vi "GUI_Highland.vi"() -> ()   [LabVIEW 2013]
uses:
  Shared/GUI_Template/GUI_master/tcp_new_data_event.ctl
  Shared/GUI_Template/GUI_master/tcp new data cluster.ctl
panel:
  out "tcp data event":T1
  in  "localsavingpath::1":path caption="LocalSavingPath"
  in  "channel4.width::1":dbl caption="Channel4.Width" min=0.0 max=10.0
  in  "channel4.delay::1":dbl caption="Channel4.Delay" min=0.0 max=10.0
  in  "channel4.polarity::1":enum16{"Direct", "Inverted"}(ring) caption="Channel4.Polarity"
  in  "channel4.channelon::1":enum16{"off", "on"}(ring) caption="Channel4.ChannelOn"
  in  "channel3.width::1":dbl caption="Channel3.Width" min=0.0 max=10.0
  in  "channel3.delay::1":dbl caption="Channel3.Delay" min=0.0 max=10.0
  in  "channel3.polarity::1":enum16{"Direct", "Inverted"}(ring) caption="Channel3.Polarity"
  in  "channel3.channelon::1":enum16{"off", "on"}(ring) caption="Channel3.ChannelOn"
  in  "channel2.width::1":dbl caption="Channel2.Width" min=0.0 max=10.0
  in  "channel2.delay::1":dbl caption="Channel2.Delay" min=0.0 max=10.0
  in  "channel2.polarity::1":enum16{"Direct", "Inverted"}(ring) caption="Channel2.Polarity"
  in  "channel2.channelon::1":enum16{"off", "on"}(ring) caption="Channel2.ChannelOn"
  in  "channel1.width::1":dbl caption="Channel1.Width" min=0.0 max=10.0
  in  "channel1.delay::1":dbl caption="Channel1.Delay" min=0.0 max=10.0
  in  "channel1.channelon::1":enum16{"off", "on"}(ring) caption="Channel1.ChannelOn"
  in  "channel1.polarity::1":enum16{"Direct", "Inverted"}(ring) caption="Channel1.Polarity"
  in  "trigger.source::1":T2(ring)=enum."Internal 80MHz" caption="Trigger.Source"
  in  "trigger.impedance::1":enum16{"10KOhm", "50Ohms"}(ring) caption="Trigger.Impedance"
  in  "trigger.divisor::1":dbl caption="Trigger.Divisor" min=1.0 max=9999.0
  in  "trigger.level::1":dbl caption="Trigger.Level" min=0.5 max=5.0
  out "UDP error message":string caption="Device Errors"
  in  "stop":bool
  in  "GUIdevice 1":string="HighlandT564DDG_Test(MM)"
  # "Channel parameters"
  # "Trigger Parameters"
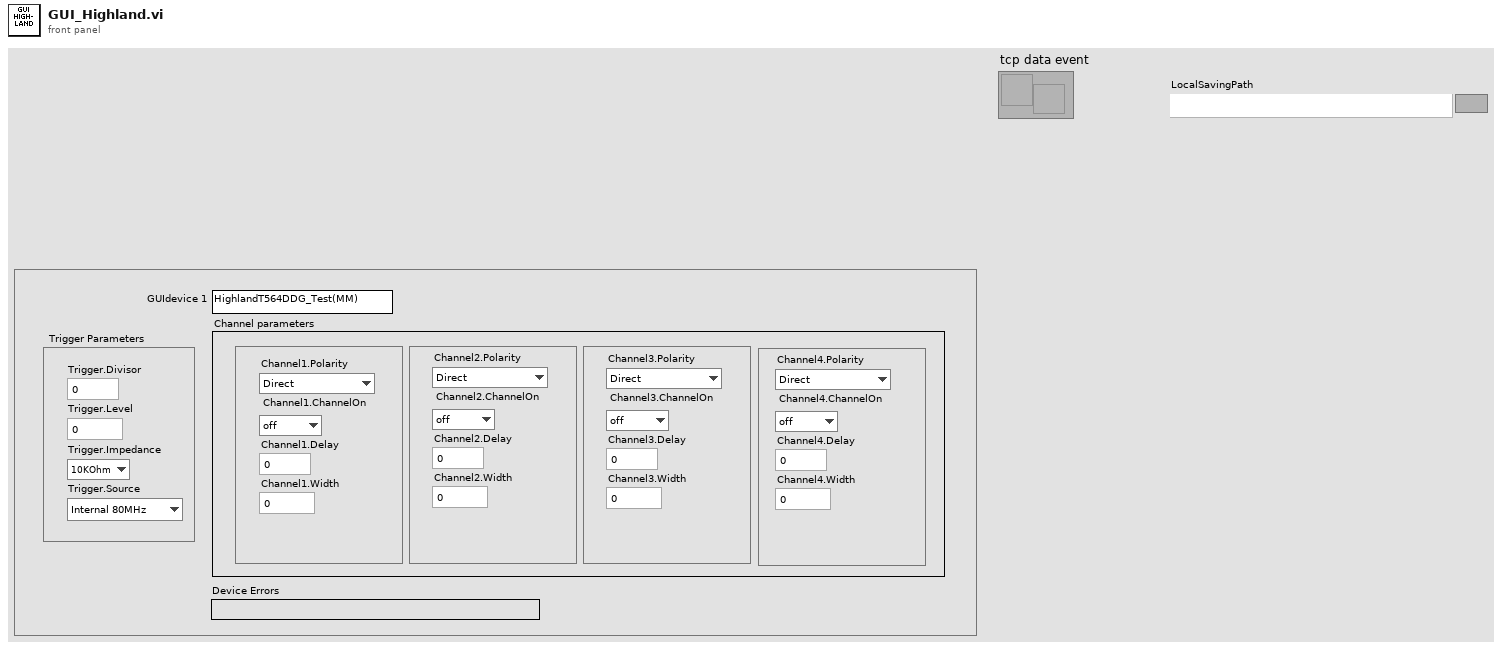
[diagram p1: front panel]
types:
  T1 = typedef "tcp_new_data_event.ctl" = refnum<user-event>
  T2 = enum16{"Rising", "Falling", "Internal 80MHz", "Internal DDS", "Remote", "Disabled"}
  T3 = enum32{"invalid app kind", "Development System", "Run Time System", "Student Edition", "Embedded LabVIEW", "Evaluation", "Custom"}
  T4 = typedef "tcp new data cluster.ctl" = cluster{"EventEnum":enum16{"new data", "connection status update"}, "Device name":string}
  T5 = enum32{"Invalid", "Standard", "Closed", "Hidden", "Minimized", "Maximized"}
  T6 = cluster{"Core":cluster{"Current VI Reference":refnum<vi>, "Close Panel on Exit?":bool}, "Your Boolean data":bool, "Your string data":string, "SuperGUI":cluster{"STOP queue":refnum<queue>, "SuperGUI ref":refnum<vi>}}
  T7 = cluster{"STOP queue":refnum<queue>, "SuperGUI ref":refnum<vi>}
  T8 = cluster{"Current VI Reference":refnum<vi>, "Close Panel on Exit?":bool}
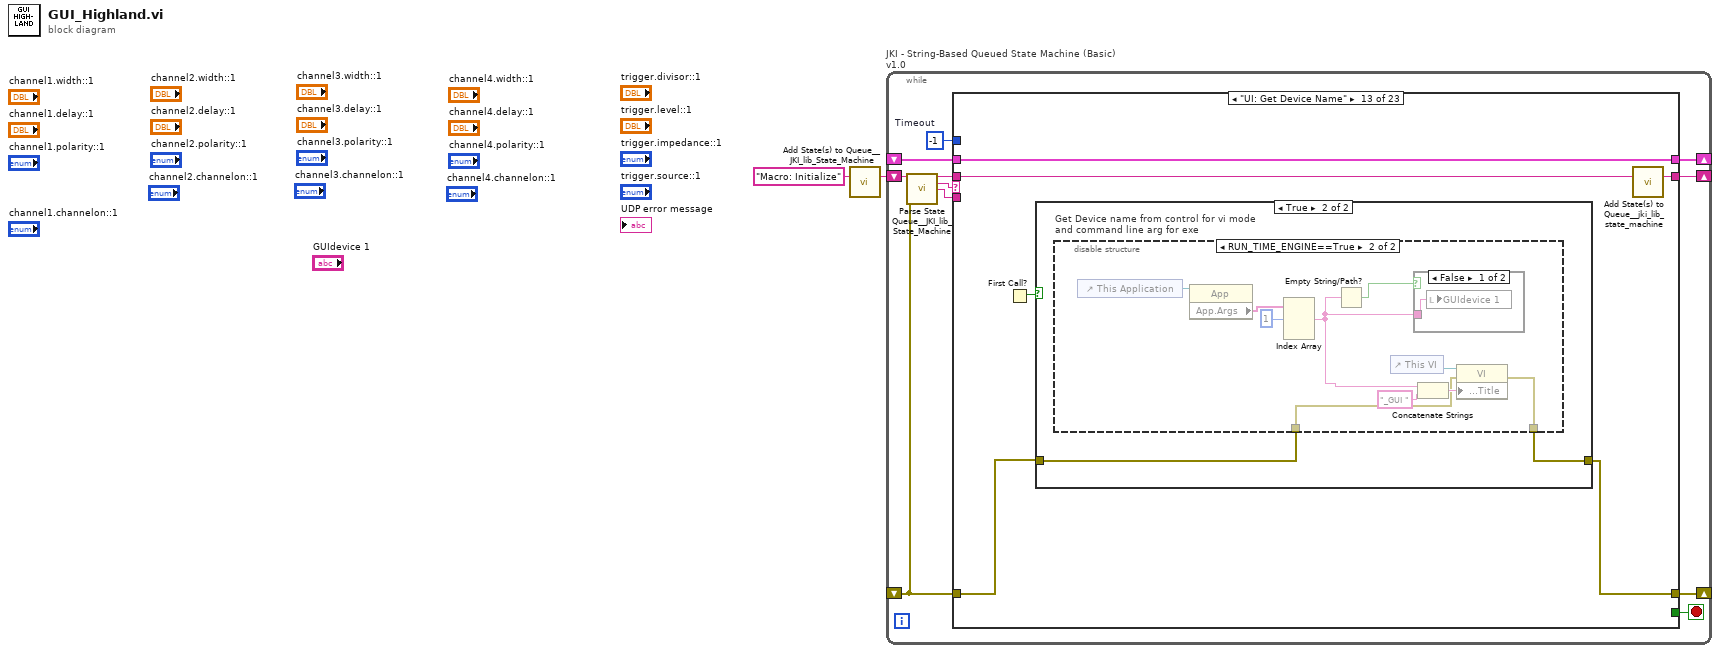
[diagram p0: block diagram]
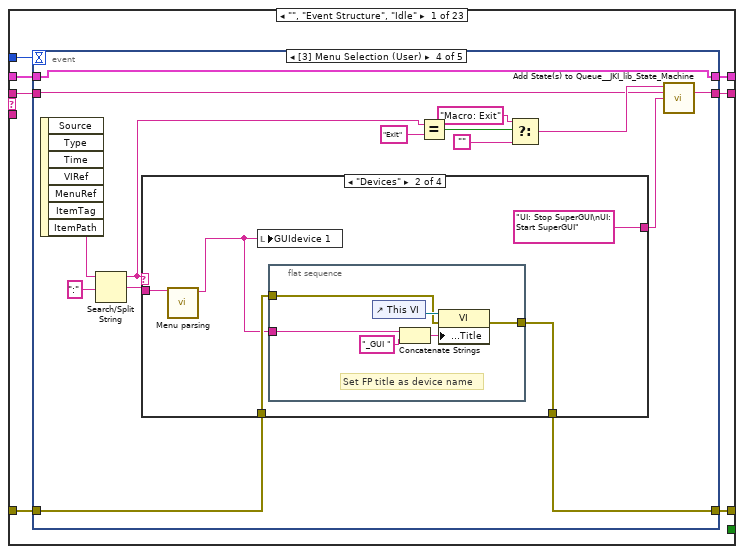
[diagram p2: hidden frame]
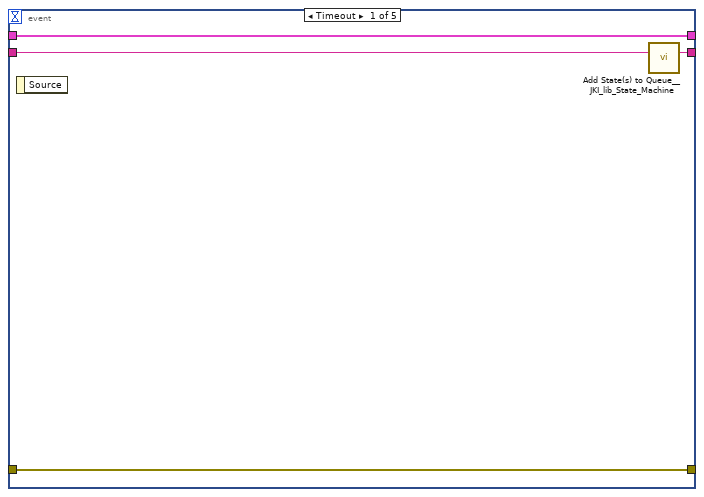
[diagram p3: hidden frame]
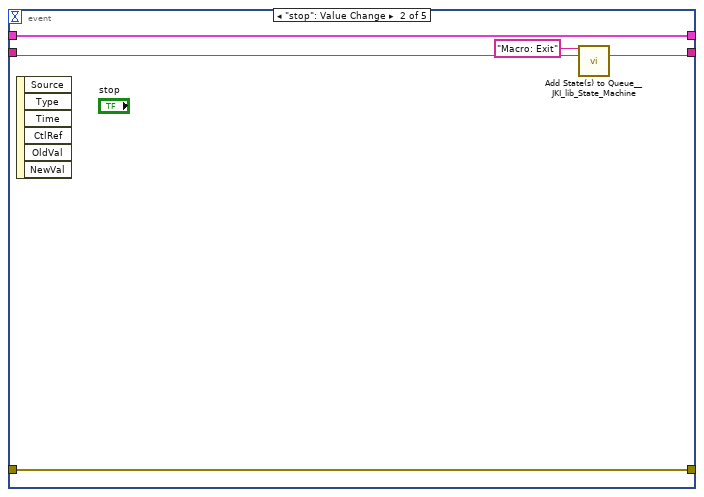
[diagram p4: hidden frame]
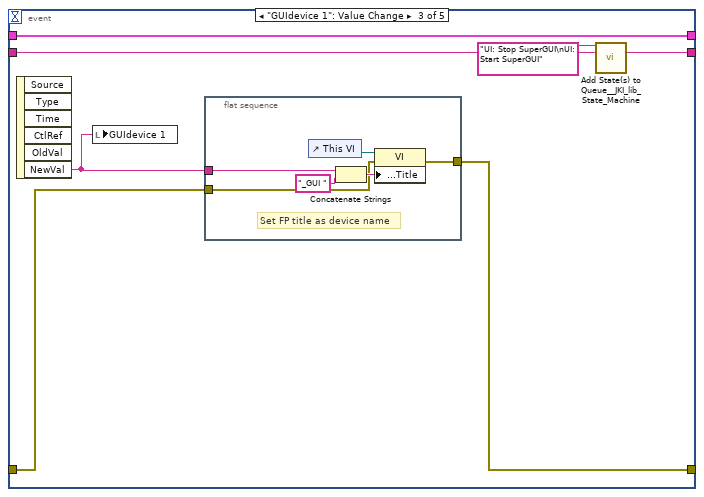
[diagram p5: hidden frame]
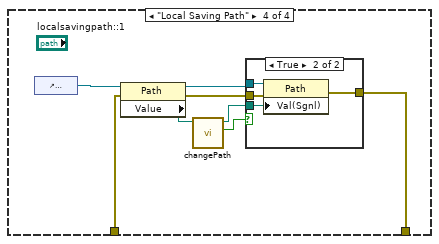
[diagram p8: hidden frame]
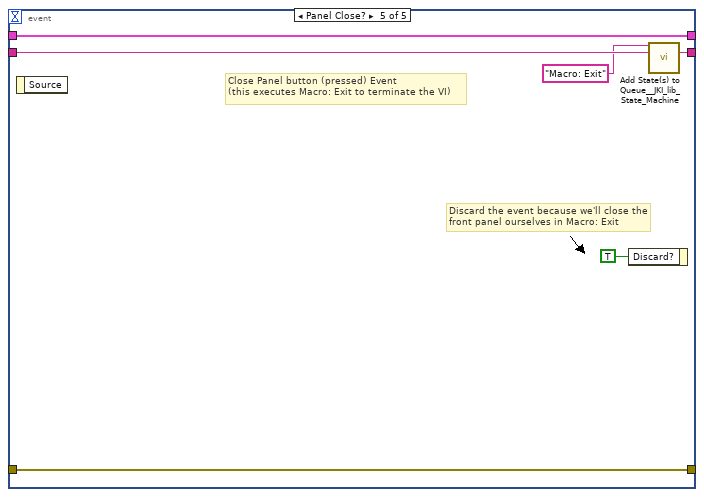
[diagram p10: hidden frame]
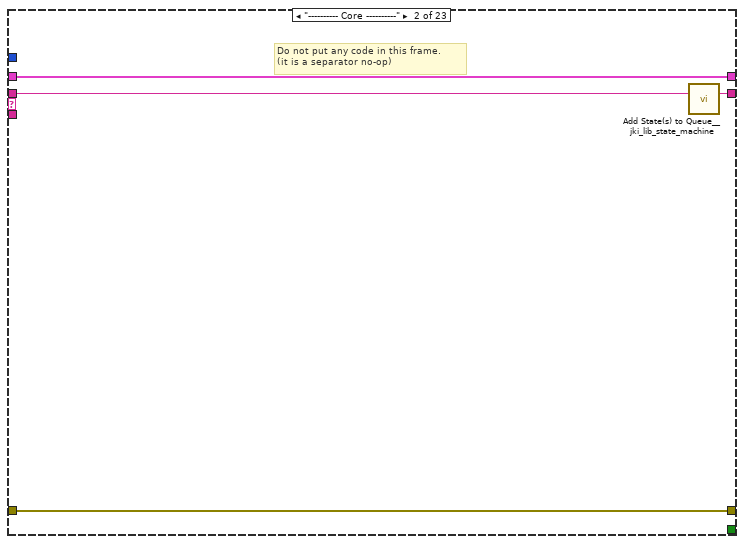
[diagram p11: hidden frame]
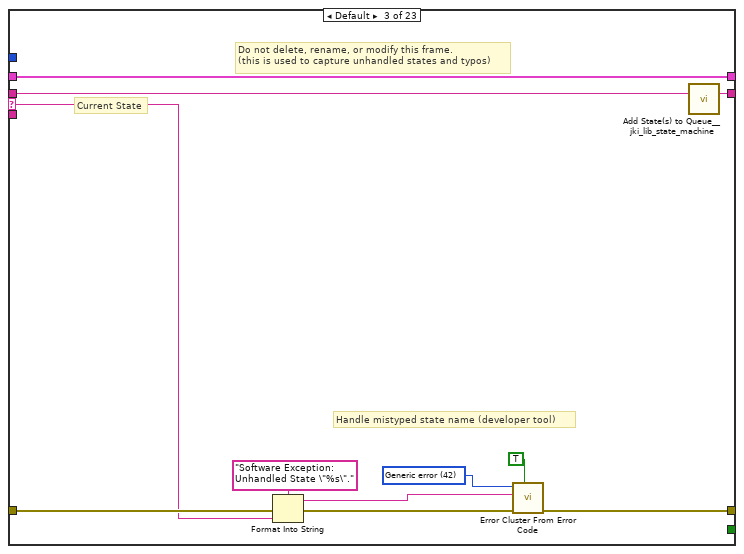
[diagram p12: hidden frame]
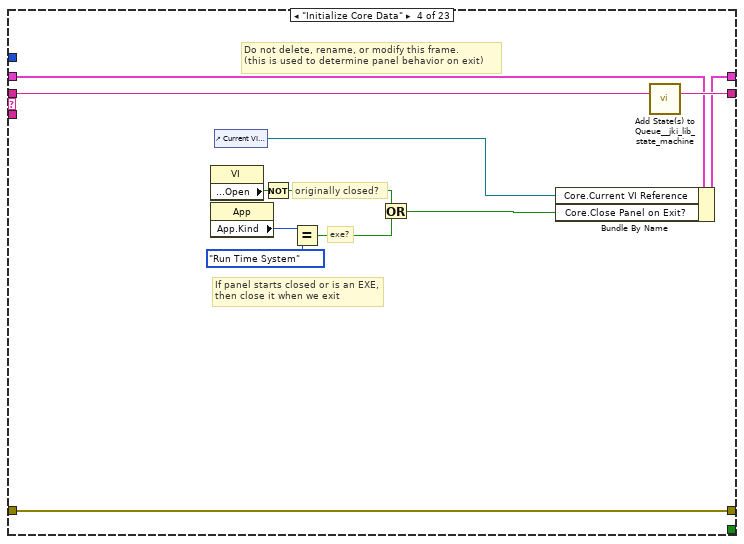
[diagram p13: hidden frame]
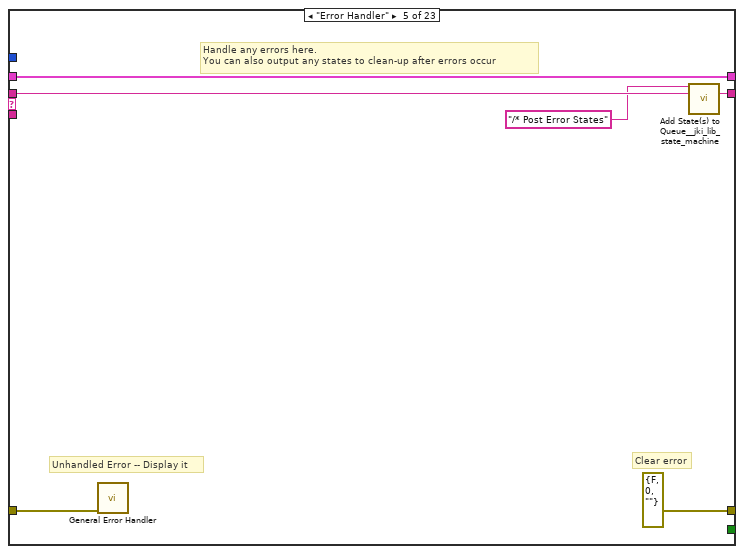
[diagram p14: hidden frame]
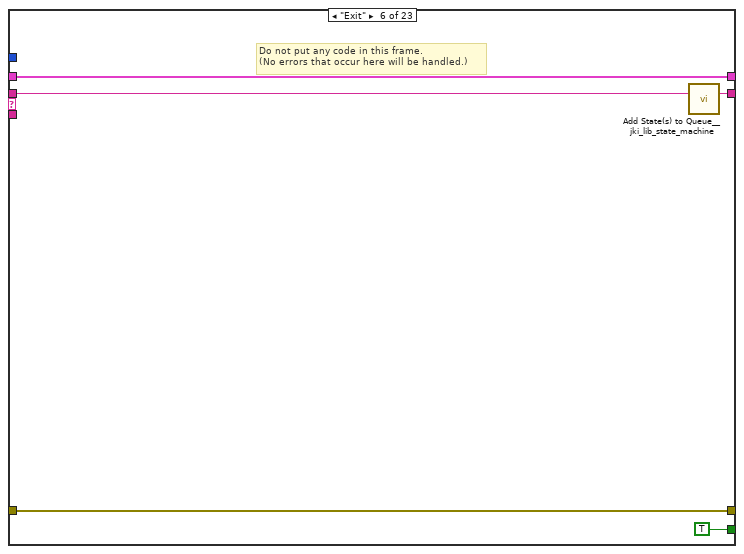
[diagram p15: hidden frame]
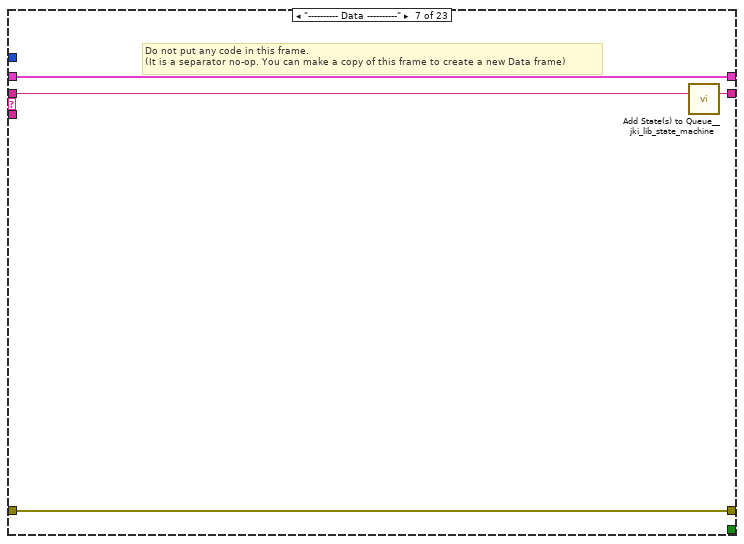
[diagram p16: hidden frame]
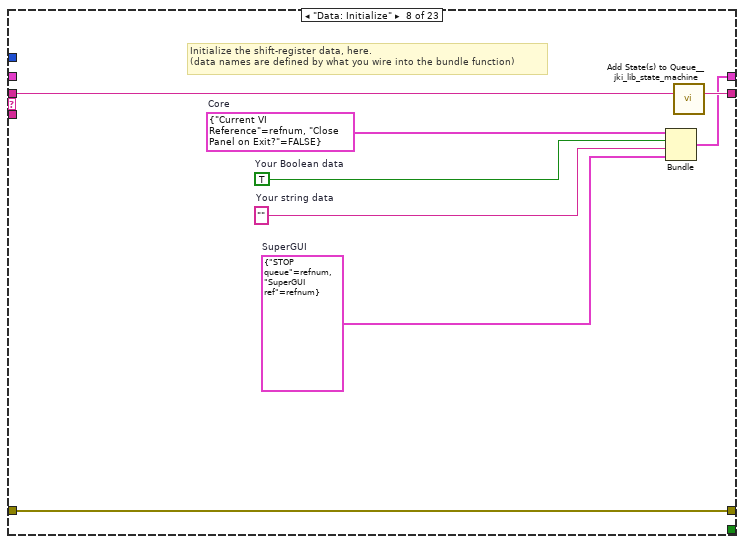
[diagram p17: hidden frame]
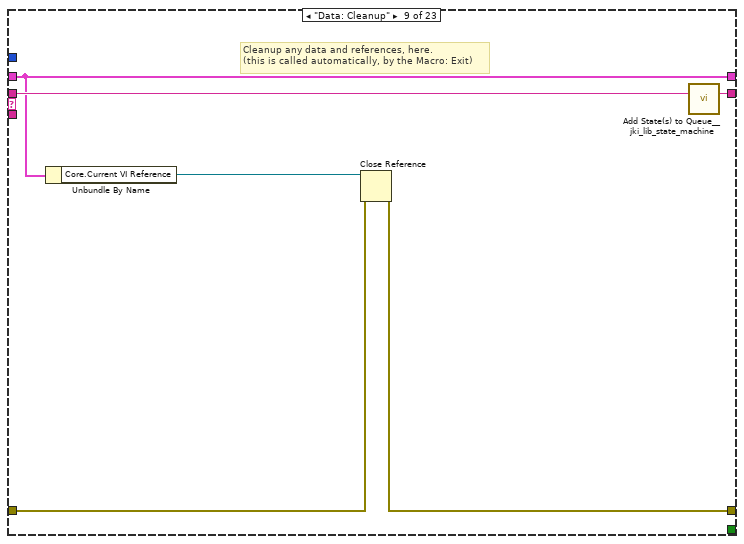
[diagram p18: hidden frame]
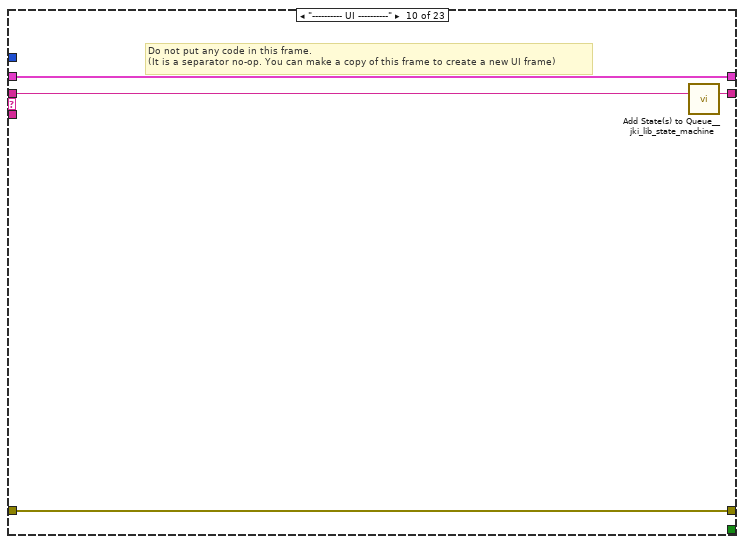
[diagram p19: hidden frame]
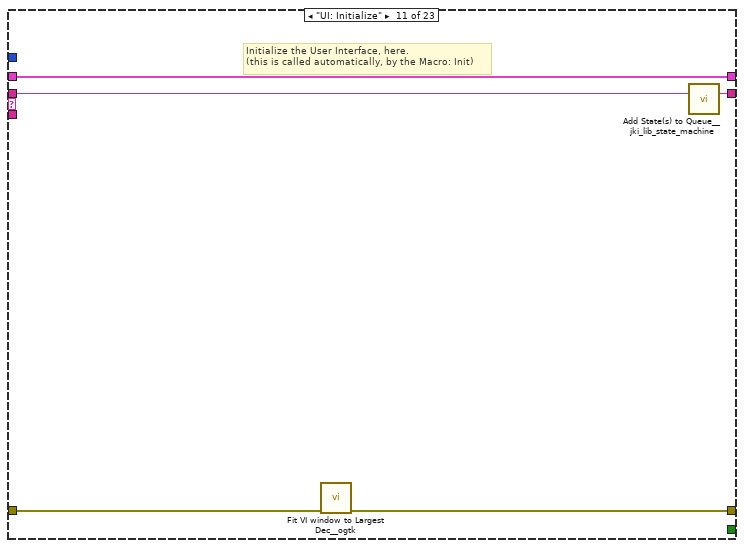
[diagram p20: hidden frame]
diagram:
  n1 = call <vilib>:"Add State(s) to Queue__JKI_lib_State_Machine.vi"("State(s) in (\"\")"="Macro: Initialize") -> ("States Out"=w2:string)  [unwired: 14 in]
  n2 = while "JKI - String-Based Queued State Machine (Basic) v1.0" {
    shift-right: [w6] -> _
    shift-left: _ -> [w5]
    shift-right: [w9] -> _
    shift-left: _ -> [w3]
    shift-right: [w8] -> _
    shift-left: w2 -> [w10]
    stop <- w7 stop-if-true
    w4 = -1  # Timeout
    n3 = call <vilib>:"Parse State Queue__JKI_lib_State_Machine.vi"("State Queue"=w10, "Error In (no error)"=w3) -> ("Remaining States"=w12:string, "Current State"=w13:string, "Arguments"=w11:string)  [unwired: 11 in]
    n4 = case shown="\"UI: Get Device Name\"" w13 {
      selector: w13 -> [_ _ w94 _ _ _ _ _ _ _ _ _ _ _ _ _ _ _ _ _ _ _ _]
      tunnel: w12 -> [w20 w93 w98 w116 w122 w127 w131 w139 w145 w149 w154 w162 w194 w228 w236 w242 w253 w279 w284 w294 w298 w302 w306]
      tunnel: w11 -> [_ _ _ _ _ _ _ _ _ _ _ _ _ _ _ w237 w247 _ _ _ _ _ _]
      tunnel: w5 -> [w18 w90 w96 w107 w119 w125 w128 _ w140 w146 w152 w160 w192 w219 w231 w240 w249 w276 w281 w291 w295 w299 w303]
      tunnel: [w17 w91 w100 w113 errorcluster {"status"=FALSE, "code"=0, "source"=""} ("error out") w124 w129 w136 w141 w147 w150 w158 w189 w212 w229 w238 w250 w277 w282 w292 w296 w300 w304] -> w9
      tunnel: w3 -> [w16 w91 w99 w113 w118 w124 w129 w136 w142 w147 w151 w159 w190 w213 w230 w239 w251 w277 w282 w292 w296 w300 w304]
      tunnel: [w19 w92 w97 w115 w121 w126 w130 w138 w144 w148 w153 w161 w193 w227 w235 w241 w252 w278 w283 w293 w297 w301 w305] -> w8
      tunnel: [_ _ _ _ _ TRUE _ _ _ _ _ _ _ _ _ _ _ _ _ _ _ _ _] -> w7
      tunnel: [w15 w90 w96 w114 w119 w125 w128 w137 w140 w146 w152 w160 w192 w218 w231 w240 w249 w276 w281 w291 w295 w299 w303] -> w6
      tunnel: w4 -> [w14 _ _ _ _ _ _ _ _ _ _ _ _ _ _ _ _ _ _ _ _ _ _]
      frame "", "Event Structure", "Idle" {
        n5 = event shown="[3] Menu Selection (User)" {
          selector: _ -> [_ _ _ _ _]
          dyn-events: _ -> [_ _ _ _ _]
          timeout: w14 -> [_ _ _ _ _]
          tunnel: w20 -> [w24 w27 w33 w51 w89]
          tunnel: [w23 w26 w32 w50 w88] -> w19
          tunnel: w18 -> [w21 w29 w36 w57 w86]
          tunnel: [w22 w28 w34 w44 w87] -> w17
          tunnel: w16 -> [w22 w28 w35 w45 w87]
          tunnel: [w21 w29 w36 w57 w86] -> w15
          event Timeout {
            n6 = event-data() -> ()  [unwired: 1 in, 1 out]
            n7 = call <vilib>:"Add State(s) to Queue__JKI_lib_State_Machine.vi"("State(s) in (\"\")"=w24) -> ("States Out"=w23:string)  [unwired: 14 in]
          }
          event "stop": Value Change {
            n8 = event-data() -> ()  [unwired: 1 in, 6 out]
            n9 = call <vilib>:"Add State(s) to Queue__JKI_lib_State_Machine.vi"("State(s) in Front (\"\")"="Macro: Exit", "State(s) in (\"\")"=w27) -> ("States Out"=w26:string)  [unwired: 13 in]
          }
          event "GUIdevice 1": Value Change {
            n10 = event-data() -> ("NewVal"=w30:string)  [unwired: 1 in, 5 out]
            n11 = local write "GUIdevice 1"(w30) -> ()
            n12 = flat-sequence {
              tunnel: [w39] -> w34
              tunnel: w35 -> [w38]
              tunnel: w30 -> [w37]
              frame #0 {
                # "Set FP title as device name"
                n13 = control-ref of="This VI"() -> (w42:refnum<vi>)
                n14 = Concatenate Strings(w37, "_GUI ") -> (w41:string)
                n15 = property class="VI"(reference=w42, error in=w38, "Front Panel.Title"=w41) -> (error out=w39:errorcluster)  [unwired: 1 out]
              }
            }
            n16 = call <vilib>:"Add State(s) to Queue__JKI_lib_State_Machine.vi"("State(s) in Front (\"\")"="UI: Stop SuperGUI\nUI: Start SuperGUI", "State(s) in (\"\")"=w33) -> ("States Out"=w32:string)  [unwired: 13 in]
          }
          event Menu Selection (User) {
            n17 = event-data() -> ("ItemPath"=w47:string)  [unwired: 1 in, 6 out]
            n18 = Search/Split String(string=w47, search string/char (-)=":") -> (substring before match=w43:string, match + rest of string=w46:string)  [unwired: 1 in, 1 out]
            n19 = case shown="\"Devices\"" w43 {
              tunnel: w46 -> [_ w63 _ _]
              tunnel: w45 -> [w58 w62 w70 w73]
              tunnel: [w58 w61 w70 w72] -> w44
              tunnel: [_ "UI: Stop SuperGUI\nUI: Start SuperGUI" _ _] -> w49
              frame "", Default {
              }
              frame "Devices" {
                n20 = call "Menu parsing.vi"("ItemPath"=w63) -> ("ItemPath"=w59:string)  [unwired: 9 in, 1 out]
                n21 = local write "GUIdevice 1"(w59) -> ()
                n22 = flat-sequence {
                  tunnel: [w66] -> w61
                  tunnel: w62 -> [w65]
                  tunnel: w59 -> [w64]
                  frame #0 {
                    # "Set FP title as device name"
                    n23 = control-ref of="This VI"() -> (w69:refnum<vi>)
                    n24 = Concatenate Strings(w64, "_GUI ") -> (w68:string)
                    n25 = property class="VI"(reference=w69, error in=w65, "Front Panel.Title"=w68) -> (error out=w66:errorcluster)  [unwired: 1 out]
                  }
                }
              }
              frame "Exit" {
              }
              frame "Local Saving Path" {
                n26 = control-ref of="localsavingpath::1"() -> (w74:refnum<vi>)
                n27 = property class="Path"(reference=w74, error in=w73) -> (reference out=w76:refnum<vi>, error out=w71:errorcluster, "Value"=w75:path)
                n28 = call "changePath.vi"("Local Saving in (h)"=w75) -> ("change (h)"=w77:bool, "Local Saving out (h)"=w78:path)  [unwired: 9 in]
                n29 = case shown="True" w77 {
                  tunnel: w76 -> [_ w83]
                  tunnel: w78 -> [_ w82]
                  tunnel: [w79 w81] -> w72
                  tunnel: w71 -> [w79 w80]
                  frame False {
                  }
                  frame True {
                    n30 = property class="Path"(reference=w83, error in=w80, "Val(Sgnl)"=w82) -> (error out=w81:errorcluster)  [unwired: 1 out]
                  }
                }
              }
            }
            n31 = Equal?(x=w43, y="Exit") -> (x = y?=w55:bool)
            n32 = Select(t="Macro: Exit", s=w55, f="") -> (s? t:f=w52:string)
            n33 = call <vilib>:"Add State(s) to Queue__JKI_lib_State_Machine.vi"("State(s) in Front (\"\")"=w52, "State(s) in (\"\")"=w51, "State(s) at Back (\"\")"=w49) -> ("States Out"=w50:string)  [unwired: 12 in]
          }
          event Panel Close? {
            # "Discard the event because we'll close the front panel ourselves in Macro: Exit"
            # "Close Panel button (pressed) Event\n(this executes Macro: Exit to terminate the VI)"
            n34 = event-data() -> ()  [unwired: 1 in, 1 out]
            n35 = event-data("Discard?"=TRUE) -> ()  [unwired: 1 in, 1 out]
            n36 = call <vilib>:"Add State(s) to Queue__JKI_lib_State_Machine.vi"("State(s) in Front (\"\")"="Macro: Exit", "State(s) in (\"\")"=w89) -> ("States Out"=w88:string)  [unwired: 13 in]
          }
        }
      }
      frame "---------- Core ----------" {
        # "Do not put any code in this frame.\n(it is a separator no-op)"
        n37 = call <vilib>:"Add State(s) to Queue__jki_lib_state_machine.vi"("State(s) in (\"\")"=w93) -> ("States Out"=w92:string)  [unwired: 14 in]
      }
      frame Default {
        w103 = 42 items=["No error", "Argument error", "Memory is full", "Out of zone", "End of file", "File already open", "Generic file I/O error", "File not found", "File permission error", "Disk is full", "Duplicate path", "Too many files open", "System feature not enabled", "Resource file not found", "Cannot add resource", "Resource not found", "Image not found", "Image memory error", "Pen does not exist", "Config type invalid", "Config token not found", "Config parse error", "Config memory error", "Bad external code format", "Bad external code offset", "External code not present", "Null window", "Destroy window error", "Null menu", "Print aborted", "Bad print record", "Print driver error", "Windows error during printing", "Memory error during printing", "Print dialog error", "Generic print error", "Invalid device refnum", "Device not found", "Device parameter error", "Device unit error", "Cannot open device", "Device call aborted", "Generic error", "Cancelled by user", "Object ID too low", "Object ID too high", "Object not in heap", "Unknown heap", "Unknown object (invalid DefProc)", "Unknown object (DefProc not in table)", "Message out of range", "Invalid (null) method", "Unknown message", "Manager call not supported", "Bad address", "Network operation in progress", "Network operation timed out", "Connection is busy", "Network attribute not supported", "Network error", "Address in use", "System out of memory", "Connection aborted", "Connection refused", "Not connected", "Already connected", "Connection closed", "Initialization error (interapplication manager)", "Bad occurrence", "Wait on unbound occurrence handler", "Occurrence queue overflow", "Datalog type conflict", "Unused", "Unrecognized type (interapplication manager)", "Memory corrupt", "Failed to make temporary DLL", "Old CIN version", "Drag socket not found", "Failed to load drop-object", "Failed to register OLE object", "Failed to release OLE object", "Format specifier type mismatch", "Unknown format specifier", "Too few format specifiers", "Too many format specifiers", "Scan failed", "Newer CIN version", "Error converting to variant", "Runtime menu error", "Password tampered", "Variant attribute not found", "Incompatible variant data type", "Event data is not available", "Event Store is not present", "Occurrence is not found", "Event Queue is not created", "Event info is not available", "Refnum passed is NULL", "Error retrieving Class GUID", "Error retrieving CoClass GUID", "Error retrieving TypeLib GUID.", "Bad built application magic bytes.", "Specific driver is different from the specific driver associated with the Logical Name.", "There is no session opened to the class driver.", "Max Error", "MAX - Error with config objects", "MAX - Error loading configuration", "MAX - Group not supported"]
        # "Current State"
        # "Do not delete, rename, or modify this frame.\n(this is used to capture unhandled states and typos)"
        # "Handle mistyped state name (developer tool)"
        n38 = Format Into String(format string="Software Exception: Unhandled State \"%s\"." ("message"), error in=w99, w94) -> (resulting string=w102:string, error out=w101:errorcluster)  [unwired: 1 in]
        n39 = call <vilib>:"Error Cluster From Error Code.vi"("show call chain? (False)"=TRUE, "error in (no error)"=w101, "error message (\"\")"=w102, "error code (0)"=w103) -> ("error out"=w100:errorcluster)  [unwired: 5 in]
        n40 = call <vilib>:"Add State(s) to Queue__jki_lib_state_machine.vi"("State(s) in (\"\")"=w98) -> ("States Out"=w97:string)  [unwired: 14 in]
      }
      frame "Initialize Core Data" {
        # "Do not delete, rename, or modify this frame.\n(this is used to determine panel behavior on exit)"
        # "originally closed?"
        # "exe?"
        # "If panel starts closed or is an EXE, then close it when we exit"
        n41 = property class="VI"() -> ("Front Panel.Open"=w112:bool)  [unwired: 2 in, 2 out]
        n42 = property class="App"() -> ("App.Kind"=w111:T3)  [unwired: 2 in, 2 out]
        n43 = control-ref of="Current VI Reference"() -> (w105:refnum<vi>)
        n44 = Not(x=w112) -> (.not. x?=w109:bool)
        n45 = Equal?(x=w111, y=T3."Run Time System" ("Application:Kind")) -> (x = y?=w108:bool)
        n46 = Or(x=w109, y=w108) -> (x .or. y?=w106:bool)
        n47 = Bundle By Name(cluster=w107, "Core.Current VI Reference"=w105, "Core.Close Panel on Exit?"=w106) -> (w114:T6)
        n48 = call <vilib>:"Add State(s) to Queue__jki_lib_state_machine.vi"("State(s) in (\"\")"=w116) -> ("States Out"=w115:string)  [unwired: 14 in]
      }
      frame "Error Handler" {
        # "Unhandled Error -- Display it"
        # "Handle any errors here.\nYou can also output any states to clean-up after errors occur"
        # "Clear error"
        n49 = call <vilib>:"General Error Handler.vi"("error in (no error)"=w118) -> ()  [unwired: 10 in, 5 out]
        n50 = call <vilib>:"Add State(s) to Queue__jki_lib_state_machine.vi"("State(s) in Front (\"\")"="/* Post Error States", "State(s) in (\"\")"=w122) -> ("States Out"=w121:string)  [unwired: 13 in]
      }
      frame "Exit" {
        # "Do not put any code in this frame.\n(No errors that occur here will be handled.)"
        n51 = call <vilib>:"Add State(s) to Queue__jki_lib_state_machine.vi"("State(s) in (\"\")"=w127) -> ("States Out"=w126:string)  [unwired: 14 in]
      }
      frame "---------- Data ----------" {
        # "Do not put any code in this frame.\n(It is a separator no-op. You can make a copy of this frame to create a new Data frame)"
        n52 = call <vilib>:"Add State(s) to Queue__jki_lib_state_machine.vi"("State(s) in (\"\")"=w131) -> ("States Out"=w130:string)  [unwired: 14 in]
      }
      frame "Data: Initialize" {
        w132 = T7 {"STOP queue"=refnum, "SuperGUI ref"=refnum}  # SuperGUI
        w133 = T8 {"Current VI Reference"=refnum, "Close Panel on Exit?"=FALSE}  # Core
        w135 = TRUE  # Your Boolean data
        w134 = ""  # Your string data
        # "Initialize the shift-register data, here.\n(data names are defined by what you wire into the bundle function)"
        n53 = Bundle("Core"=w133, "Your Boolean data"=w135, "Your string data"=w134, "SuperGUI"=w132) -> (w137:T6)  [unwired: 1 in]
        n54 = call <vilib>:"Add State(s) to Queue__jki_lib_state_machine.vi"("State(s) in (\"\")"=w139) -> ("States Out"=w138:string)  [unwired: 14 in]
      }
      frame "Data: Cleanup" {
        # "Cleanup any data and references, here.\n(this is called automatically, by the Macro: Exit)"
        n55 = Unbundle By Name(w140) -> ("Core.Current VI Reference"=w143:refnum<vi>)
        n56 = Close Reference(reference=w143, error in (no error)=w142) -> (error out=w141:errorcluster)
        n57 = call <vilib>:"Add State(s) to Queue__jki_lib_state_machine.vi"("State(s) in (\"\")"=w145) -> ("States Out"=w144:string)  [unwired: 14 in]
      }
      frame "---------- UI ----------" {
        # "Do not put any code in this frame.\n(It is a separator no-op. You can make a copy of this frame to create a new UI frame)"
        n58 = call <vilib>:"Add State(s) to Queue__jki_lib_state_machine.vi"("State(s) in (\"\")"=w149) -> ("States Out"=w148:string)  [unwired: 14 in]
      }
      frame "UI: Initialize" {
        # "Initialize the User Interface, here.\n(this is called automatically, by the Macro: Init)"
        n59 = call <userlib>:"Fit VI window to Largest Dec__ogtk.vi"("error in (no error)"=w151) -> ("error out"=w150:errorcluster)  [unwired: 5 in, 1 out]
        n60 = call <vilib>:"Add State(s) to Queue__jki_lib_state_machine.vi"("State(s) in (\"\")"=w154) -> ("States Out"=w153:string)  [unwired: 14 in]
      }
      frame "UI: Update Device List" {
        n61 = call "getDevices.vi"("Device Class"="Highland T564 DDG") -> ("All Devices"=w156:string[])
        n62 = Empty Array?(array=w156) -> (empty?=w157:bool)
        n63 = case shown="False" w157 {
          tunnel: w159 -> [w165 w188]
          tunnel: [w164 w188] -> w158
          tunnel: w156 -> [w163 _]
          frame False {
            n64 = Current VI's Menubar() -> (w168:refnum<k9>)
            n65 = Get Menu Item Info(7:"Devices" ("item tag"), 8:w165, 11:w168) -> (0:w174:errorcluster, 3:w170:refnum<k9>)  [unwired: 5 out]
            n66 = Set Menu Item Info(7:"Devices" ("item tag"), 8:w174, 9:TRUE ("enabled"), 11:w170) -> (0:w173:errorcluster, 3:w172:refnum<k9>)  [unwired: 3 in]
            n67 = First Call?() -> (First Call?: T/F=w166:bool)
            n68 = case shown="True" w166 {
              tunnel: w172 -> [_ w180]
              tunnel: w163 -> [_ w179]
              tunnel: w173 -> [w175 w177]
              tunnel: [w175 w176] -> w164
              frame False {
              }
              frame True {
                n69 = for {
                  tunnel: [w187] -> w181
                  tunnel: w179 -> [w185] mode=indexing
                  tunnel: w180 -> [w184]
                  tunnel: [w183] -> w178
                  tunnel: w177 -> [w182]
                  n70 = Insert Menu Items(5:"Devices" ("menu tag"), 6:w182, 7:w185, 8:w185, 9:w184) -> (0:w183:errorcluster, 3:w187:refnum<k9>)  [unwired: 1 in, 1 out]
                }
                n71 = Enable Menu Tracking(2:w178, 4:w181) -> (0:w176:errorcluster)  [unwired: 1 in, 1 out]
              }
            }
          }
          frame True {
          }
        }
        n72 = call <vilib>:"Add State(s) to Queue__jki_lib_state_machine.vi"("State(s) in (\"\")"=w162) -> ("States Out"=w161:string)  [unwired: 14 in]
      }
      frame "UI: Get Device Name" {
        n73 = First Call?() -> (First Call?: T/F=w191:bool)
        n74 = case shown="True" w191 {
          tunnel: w190 -> [w195 w197]
          tunnel: [w195 w196] -> w189
          frame False {
          }
          frame True {
            n75 = disable-structure "Get Device name from control for vi mode\nand command line arg for exe" shown="RUN_TIME_ENGINE==True" {
              disable-tunnel: w197 -> [_ w199]
              disable-tunnel: [_ w198] -> w196
              frame condition #0 (active) {
              }
              frame condition #1 {
                n76 = control-ref of="This Application"() -> (w207:refnum<vi>)
                n77 = property class="App"(reference=w207) -> ("App.Args"=w206:string[])  [unwired: 1 in, 2 out]
                n78 = Index Array(array=w206, index #1=1 ("index")) -> (element #1=w200:string)  [unwired: 2 in, 2 out]
                n79 = Empty String/Path?(string/path=w200) -> (empty?=w204:bool)
                n80 = control-ref of="This VI"() -> (w203:refnum<vi>)
                n81 = case shown="False" w204 {
                  tunnel: w200 -> [w208 _]
                  frame False {
                    n82 = local write "GUIdevice 1"(w208) -> ()
                  }
                  frame True {
                  }
                }
                n83 = Concatenate Strings(w200, "_GUI ") -> (w202:string)
                n84 = property class="VI"(reference=w203, error in=w199, "Front Panel.Title"=w202) -> (error out=w198:errorcluster)  [unwired: 1 out]
              }
            }
          }
        }
        n85 = call <vilib>:"Add State(s) to Queue__jki_lib_state_machine.vi"("State(s) in (\"\")"=w194) -> ("States Out"=w193:string)  [unwired: 14 in]
      }
      frame "UI: Start SuperGUI" {
        # "create stop queue for supergui and its clones"
        # "x100 abort will be dependent on caller VI\nx80 abort will be independent of caller vi, this will abort vi when labview is closed."
        # "Start SuperGUI asynchronous way"
        n86 = vi-ref "GUI_Master_subvi_reentrant_queues.vi"() -> (w211:refnum<vi>)
        n87 = property class="VI"(reference=w211) -> ("Path"=w210:path)  [unwired: 1 in, 2 out]
        n88 = Create User Event(user event datatype=T4 {"EventEnum"=enum."new data", "Device name"="Device name"} ("New Event"), error in=w213) -> (user event=w214:refnum<user-event>, error out=w220:errorcluster)
        "tcp data event" <- w214
        n89 = control-ref of="This Application"() -> (w217:refnum<vi>)
        n90 = control-ref of="This VI"() -> (w216:refnum<vi>)
        n91 = Open VI Reference(type specifier VI Refnum (for type only)=refnum<vi> refnum, vi path=w210, options=256) -> (vi reference=w226:refnum<vi>, error out=w225:errorcluster)  [unwired: 3 in]
        n92 = register-events(w214) -> ()  [unwired: 2 in, 2 out]
        n93 = call "supergui create stop queue.vi"() -> ("STOP Queue out"=w222:refnum<queue>)  [unwired: 11 in]
        n94 = Current VI's Menubar() -> (w215:refnum<k9>)
        n95 = call-by-ref "Start Asynchronous Call"(reference=w226, error in=w225, "STOP Queue in"=w222, "This Application"=w217, 8:"error in (no error)"=w220, "tcp data event"=w214, "Caller menu reference"=w215, "Caller VI ref"=w216) -> (reference out=w209:refnum<vi>, error out=w212:errorcluster)  [unwired: 5 in, 1 out]
        n96 = Bundle By Name(cluster=w219, "SuperGUI.SuperGUI ref"=w209, "SuperGUI.STOP queue"=w222) -> (w218:T6)
        n97 = call <vilib>:"Add State(s) to Queue__jki_lib_state_machine.vi"("State(s) in (\"\")"=w228) -> ("States Out"=w227:string)  [unwired: 14 in]
      }
      frame "UI: Stop SuperGUI" {
        # "Stop Supergui Clone and wait until it exit properly"
        n98 = Unbundle By Name(w231) -> ("SuperGUI.SuperGUI ref"=w233:refnum<vi>, "SuperGUI.STOP queue"=w232:refnum<queue>)
        n99 = Release Queue(queue=w232, error in (no error)=w230) -> (error out=w234:errorcluster)  [unwired: 1 in, 2 out]
        n100 = call-by-ref "Wait On Asynchronous Call"(reference=w233, error in=w234) -> ("error out"=w229:errorcluster)  [unwired: 11 in, 2 out]
        n101 = call <vilib>:"Add State(s) to Queue__jki_lib_state_machine.vi"("State(s) in (\"\")"=w236) -> ("States Out"=w235:string)  [unwired: 14 in]
      }
      frame "UI: Cursor Set" {
        # "Argument"
        # "Set and Unset Cursor Busy.\n(Usage: \"UI: Cursor Set >> Busy|Idle\")"
        n102 = case shown="\"Idle\", Default" w237 {
          tunnel: w239 -> [w244 w246]
          tunnel: [w243 w245] -> w238
          frame "Idle", Default {
            n103 = call <vilib>:"Unset Busy.vi"("error in (no error)"=w244) -> ("error out"=w243:errorcluster)  [unwired: 10 in]
          }
          frame "Busy" {
            n104 = call <vilib>:"Set Busy.vi"("error in (no error)"=w246) -> ("error out"=w245:errorcluster)  [unwired: 9 in, 1 out]
          }
        }
        n105 = call <vilib>:"Add State(s) to Queue__jki_lib_state_machine.vi"("State(s) in (\"\")"=w242) -> ("States Out"=w241:string)  [unwired: 14 in]
      }
      frame "UI: Front Panel State" {
        # "Argument"
        # "Set Front Panel Open or Closed\n(Usage: \"UI: Front Panel State >> Open|Close\")"
        n106 = Unbundle By Name(w249) -> ("Core.Current VI Reference"=w248:refnum<vi>)
        n107 = case shown="\"Open\", Default" w247 {
          tunnel: w251 -> [w257 w270]
          tunnel: [w259 w271] -> w250
          tunnel: w248 -> [w258 w268]
          frame "Open", Default {
            n108 = property class="VI"(reference=w258, error in=w257) -> (reference out=w255:refnum<vi>, error out=w256:errorcluster, "Front Panel.Open"=w254:bool)
            n109 = case shown="False" w254 {
              tunnel: [w262 w265] -> w259
              tunnel: w256 -> [w261 w265]
              tunnel: w255 -> [w260 _]
              frame False {
                n110 = invoke class="VI" method="FP.Open"(reference=w260, error in=w261, "Activate"=TRUE, "State"=T5."Standard") -> (error out=w262:errorcluster)  [unwired: 1 in, 4 out]
              }
              frame True {
              }
            }
          }
          frame "Close" {
            n111 = property class="VI"(reference=w268, error in=w270) -> (reference out=w267:refnum<vi>, error out=w269:errorcluster, "Front Panel.Open"=w266:bool)
            n112 = case shown="True" w266 {
              tunnel: [w272 w275] -> w271
              tunnel: w269 -> [w272 w274]
              tunnel: w267 -> [_ w273]
              frame False {
              }
              frame True {
                n113 = invoke class="VI" method="FP.Close"(reference=w273, error in=w274) -> (error out=w275:errorcluster)  [unwired: 1 in, 2 out]
              }
            }
          }
        }
        n114 = call <vilib>:"Add State(s) to Queue__jki_lib_state_machine.vi"("State(s) in (\"\")"=w253) -> ("States Out"=w252:string)  [unwired: 14 in]
      }
      frame "---------- Macro ----------" {
        # "Do not put any code in this frame.\n(It is a separator no-op. You can make a copy of this frame to create a new Macro frame)"
        n115 = call <vilib>:"Add State(s) to Queue__jki_lib_state_machine.vi"("State(s) in (\"\")"=w279) -> ("States Out"=w278:string)  [unwired: 14 in]
      }
      frame "Macro: Initialize" {
        # "Initialization Macro\n(This is called once, when the VI starts)"
        n116 = call <vilib>:"Add State(s) to Queue__jki_lib_state_machine.vi"("State(s) in Front (\"\")"="Data: Initialize\nInitialize Core Data\nUI: Initialize\nUI: Update Device List\nUI: Get Device Name\nUI: Start SuperGUI\nUI: Front Panel State >> Open", "State(s) in (\"\")"=w284) -> ("States Out"=w283:string)  [unwired: 13 in]
      }
      frame "Macro: Exit" {
        # "Exit Macro\n(This is called once, when the VI exits)"
        n117 = Unbundle By Name(w291) -> ("Core.Close Panel on Exit?"=w290:bool)
        n118 = Select(t="UI: Front Panel State >> Close", s=w290, f="") -> (s? t:f=w287:string)
        n119 = call <vilib>:"Add State(s) to Queue__jki_lib_state_machine.vi"("State(s) in (\"\")"=w287, "State(s) at Back (\"\")"="Data: Cleanup\nExit") -> ("States Out"=w285:string)  [unwired: 13 in]
        n120 = call <vilib>:"Add State(s) to Queue__jki_lib_state_machine.vi"("State(s) in Front (\"\")"=w285, "State(s) in (\"\")"=w294) -> ("States Out"=w293:string)  [unwired: 13 in]
      }
      frame "---------- New Category ----------" {
        # "Template Separator\n(You can make a copy of, or modify, this frame)"
        n121 = call <vilib>:"Add State(s) to Queue__jki_lib_state_machine.vi"("State(s) in (\"\")"=w298) -> ("States Out"=w297:string)  [unwired: 14 in]
      }
      frame "New Category: 1" {
        # "Your code here.\n(You can make a copy of, or modify, this frame)"
        n122 = call <vilib>:"Add State(s) to Queue__jki_lib_state_machine.vi"("State(s) in (\"\")"=w302) -> ("States Out"=w301:string)  [unwired: 14 in]
      }
      frame "New Category: 2" {
        # "Your code here.\n(You can make a copy of, or modify, this frame)"
        n123 = call <vilib>:"Add State(s) to Queue__jki_lib_state_machine.vi"("State(s) in (\"\")"=w306) -> ("States Out"=w305:string)  [unwired: 14 in]
      }
    }
  }
